vi "MeasurePeak.vi"(1 "address Freq":string, 4 "address LockIn":string, 5 "Freq Start":dbl, 6 "Path":path, 7 "Wait/s":dbl, 8 "Stop":dbl, 9 "Step":dbl, 10 "error in (no error) 2":errorcluster) -> (0 "String":string, 2 "Numeric":dbl, 3 "error out":errorcluster)   [LabVIEW 2010]
uses:
  <vilib>/Utility/file.llb/Write To Spreadsheet File (DBL).vi
  <vilib>/Analysis/NI_AALBase.lvlib
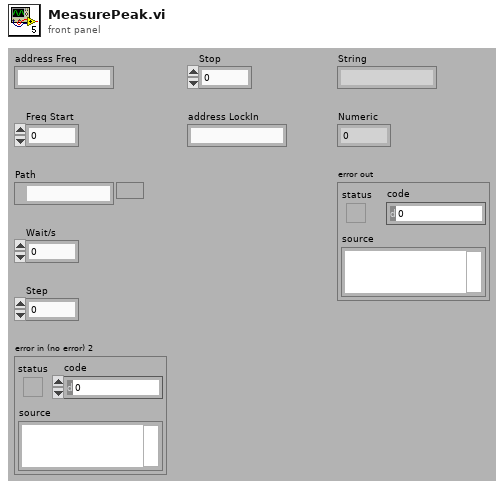
[diagram p1: front panel]
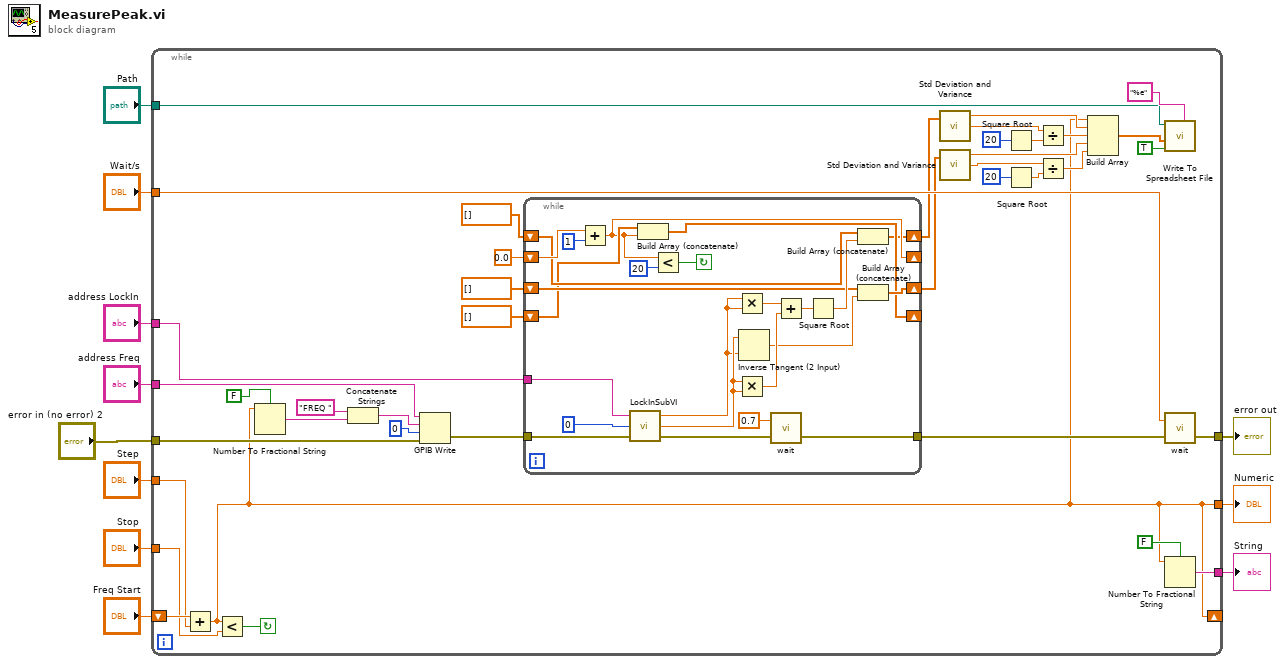
[diagram p0: block diagram]
diagram:
  n1 = while {
    tunnel: "error in (no error) 2" -> [w25]
    tunnel: [w49] -> w1
    shift-right: [w12] -> _
    shift-left: "Freq Start" -> [w19]
    tunnel: "Step" -> [w17]
    tunnel: "Stop" -> [w18]
    tunnel: "Wait/s" -> [w48]
    tunnel: "Path" -> [w32]
    tunnel: "address Freq" -> [w15]
    tunnel: [w14] -> w9
    tunnel: "address LockIn" -> [w13]
    tunnel: [w12] -> w11
    stop <- w50 continue-if-true
    n2 = Add(x=w19, y=w17) -> (x+y=w12:dbl)
    n3 = Less?(x=w12, y=w18) -> (x < y?=w50:bool)
    n4 = Number To Fractional String(use system decimal point (T)=FALSE, number=w12) -> (F-format string=w29:string)  [unwired: 2 in]
    n5 = Concatenate Strings("FREQ ", w29) -> (w28:string)
    n6 = GPIB Write(0:w15, 1:w28, 2:i16 0 ("mode (0) 2"), 3:w25) -> (6:w24:errorcluster)  [unwired: 1 in, 1 out]
    n7 = while {
      tunnel: w24 -> [w60]
      shift-right: [w55] -> _
      shift-left: 0.0 ("Start") -> [w73]
      shift-right: [w56] -> _
      shift-left: dbl[] [] -> [w57]
      shift-right: [w52] -> w37
      shift-left: dbl[] [] -> [w65]
      shift-right: [w62] -> w44
      shift-left: dbl[] [] -> [w63]
      tunnel: [w54] -> w26
      tunnel: w13 -> [w51]
      stop <- w58 continue-if-true
      n8 = Add(x=w73, y=1) -> (x+y=w55:dbl)
      n9 = call "LockInSubVI.vi"("error in"=w60, "mode (0)"=i16 0, "address string"=w51) -> ("error out 2"=w53:errorcluster, "data Y"=w68:dbl, "data X"=w67:dbl)
      n10 = Build Array (concatenate)(w57, w55) -> (w56:dbl[])
      n11 = Less?(x=w55, y=20) -> (x < y?=w58:bool)
      n12 = Multiply(x=w67, y=w67) -> (x*y=w71:dbl)
      n13 = Multiply(x=w68, y=w68) -> (x*y=w70:dbl)
      n14 = Inverse Tangent (2 Input)(1:w67, 2:w68) -> (0:w64:dbl)
      n15 = call "wait.vi"("error in"=w53, "Wartezeit in Sek"=0.7) -> ("error out"=w54:errorcluster)  [unwired: 1 in]
      n16 = Add(x=w71, y=w70) -> (x+y=w69:dbl)
      n17 = Square Root(x=w69) -> (sqrt(x)=w66:dbl)
      n18 = Build Array (concatenate)(w65, w66) -> (w52:dbl[])
      n19 = Build Array (concatenate)(w63, w64) -> (w62:dbl[])
    }
    n20 = call <vilib>:"Std Deviation and Variance.vi"("X"=w37) -> ("mean"=w21:dbl, "standard deviation"=w38:dbl)  [unwired: 1 in, 1 out]
    n21 = call <vilib>:"Std Deviation and Variance.vi"("X"=w44) -> ("mean"=w20:dbl, "standard deviation"=w41:dbl)  [unwired: 1 in, 1 out]
    n22 = Square Root(x=20) -> (sqrt(x)=w40:dbl)
    n23 = Square Root(x=20) -> (sqrt(x)=w43:dbl)
    n24 = Divide(x=w38, y=w40) -> (x/y=w16:dbl)
    n25 = Divide(x=w41, y=w43) -> (x/y=w22:dbl)
    n26 = Build Array(w12, w21, w16, w20, w22) -> (w23:dbl[])
    n27 = call-poly <vilib>:"Write To Spreadsheet File.vi"("format (%.3f)"="%e", "append to file? (new file:F)"=TRUE, "1D data"=w23, "file path (dialog if empty)"=w32) -> ()  [unwired: 4 in, 1 out]
    n28 = call "wait.vi"("error in"=w26, "Wartezeit in Sek"=w48) -> ("error out"=w49:errorcluster)  [unwired: 1 in]
    n29 = Number To Fractional String(use system decimal point (T)=FALSE, number=w12) -> (F-format string=w14:string)  [unwired: 2 in]
  }
  "Numeric" <- w11
  "String" <- w9
  "error out" <- w1
